vi "Sift Bob's Key.vi"(8 "error in":errorcluster, 10 "PM Level in":u8[](array[numeric]), 11 "SPD Number in":u8[](array[numeric])) -> (0 "error out":errorcluster, 2 "Sifted Bob's data":u32[](array[numeric]), 3 "Raw Bob's data":u8[](array[numeric]))   [LabVIEW 2018]
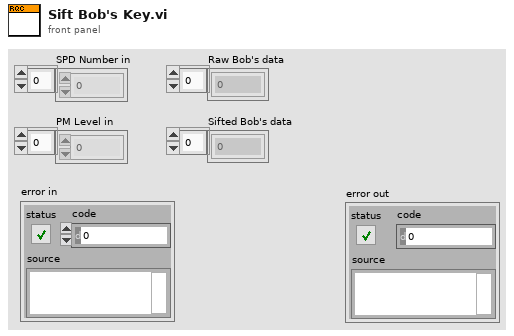
[diagram p1: front panel]
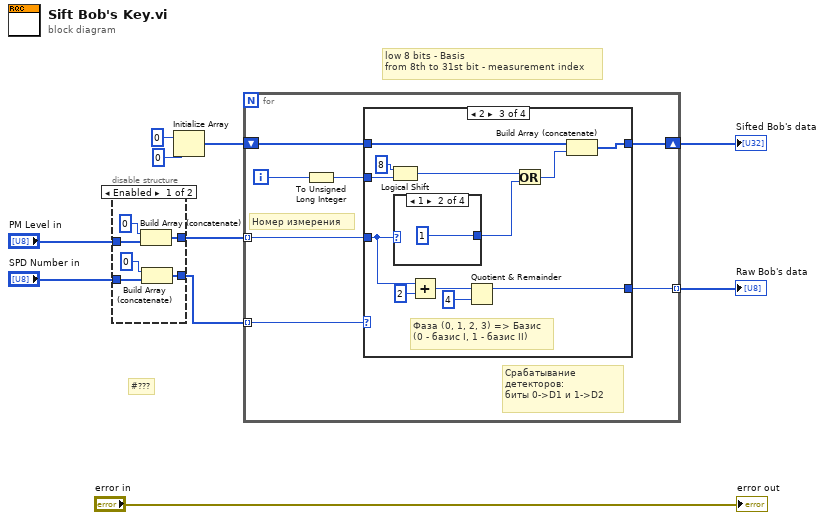
[diagram p0: block diagram]
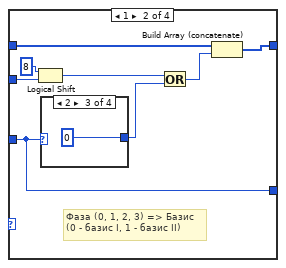
[diagram p4: hidden frame]
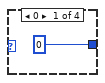
[diagram p5: hidden frame]
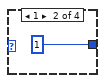
[diagram p6: hidden frame]
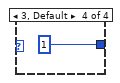
[diagram p7: hidden frame]
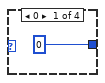
[diagram p8: hidden frame]
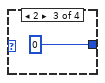
[diagram p9: hidden frame]
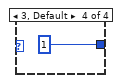
[diagram p10: hidden frame]
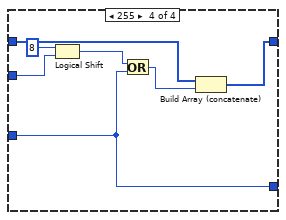
[diagram p11: hidden frame]
diagram:
  # "#???"
  # "low 8 bits - Basis\nfrom 8th to 31st bit - measurement index"
  n1 = disable-structure shown="Enabled" {
    disable-tunnel: "PM Level in" -> [w16 w18]
    disable-tunnel: [w15 w18] -> w5
    disable-tunnel: "SPD Number in" -> [w12 w17]
    disable-tunnel: [w11 w17] -> w4
    frame Enabled {
      n2 = Build Array (concatenate)(u8 0, w16) -> (w15:u8[])
      n3 = Build Array (concatenate)(u8 0, w12) -> (w11:u8[])
    }
    frame Disabled {
    }
  }
  n4 = Initialize Array(u32 0, 0 ("dimension size")) -> (w8:u32[])
  n5 = for {
    shift-right: [w25] -> w3
    shift-left: w8 -> [w24]
    tunnel: w5 -> [w22] mode=indexing
    tunnel: w4 -> [w23] mode=indexing
    tunnel: [w19] -> w2 mode=indexing
    i -> [w20]
    # "Срабатывание детекторов:\nбиты 0->D1 и 1->D2"
    # "Номер измерения"
    n6 = To Unsigned Long Integer(number=w20) -> (unsigned 32bit integer=w21:u32)
    n7 = case shown="2" w23 {
      tunnel: [w27 w32 w48 w61] -> w25
      tunnel: w24 -> [w27 w30 w46 w62]
      tunnel: w21 -> [_ w31 w47 w60]
      tunnel: w22 -> [w26 w28 w44 w56]
      tunnel: [w26 w28 w41 w56] -> w19
      frame 0, Default {
      }
      frame 1 {
        # "Фаза (0, 1, 2, 3) => Базис (0 - базис I, 1 - базис II)"
        n8 = Logical Shift(y=8, x=w31) -> (x << y=w34:u32)
        n9 = case shown="2" w28 {
          tunnel: [u32 0 u32 1 u32 0 u32 1] -> w29
          frame 0 {
          }
          frame 1 {
          }
          frame 2 {
          }
          frame 3, Default {
          }
        }
        n10 = Or(x=w34, y=w29) -> (x .or. y?=w33:u32)
        n11 = Build Array (concatenate)(w30, w33) -> (w32:u32[])
      }
      frame 2 {
        # "Фаза (0, 1, 2, 3) => Базис (0 - базис I, 1 - базис II)"
        n12 = Logical Shift(y=8, x=w47) -> (x << y=w50:u32)
        n13 = case shown="1" w44 {
          tunnel: [u32 0 u32 1 u32 0 u32 1] -> w45
          frame 0 {
          }
          frame 1 {
          }
          frame 2 {
          }
          frame 3, Default {
          }
        }
        n14 = Add(x=w44, y=u8 2) -> (x+y=w43:u8)
        n15 = Quotient & Remainder(x=w43, y=u8 4) -> (x-y*floor(x/y)=w41:u8)  [unwired: 1 out]
        n16 = Or(x=w50, y=w45) -> (x .or. y?=w49:u32)
        n17 = Build Array (concatenate)(w46, w49) -> (w48:u32[])
      }
      frame 255 {
        n18 = Logical Shift(y=8, x=w60) -> (x << y=w58:u32)
        n19 = Or(x=w58, y=w56) -> (x .or. y?=w57:u32)
        n20 = Build Array (concatenate)(w62, w57) -> (w61:u32[])
      }
    }
  }
  "Raw Bob's data" <- w2
  "Sifted Bob's data" <- w3
  "error out" <- "error in"
